vi "FTW-Logger-Construct.vi"(0 "Initialization Sequence":string, 5 "Logger Configuration":string, 11 "error in":errorcluster) -> (4 "FTW Logger":refnum<class "FTW-Logger-Core.lvclass">, 6 "Incoming Requests":refnum<event-registration>, 8 "Local Messages":refnum<event-registration>, 15 "error out":errorcluster)   [LabVIEW 2015, in "FTW-Logger-Core.lvclass"]
uses:
  FTW-Logger-Core.lvclass
  Message/Request/FTW-Message-IncomingRequest.lvclass
  Message/Base/FTW-Message.lvclass
  FTW-Logger-Core.lvclass/FTW-Logger-Core.ctl
  Error/FTW-ERR-NoErrorConstant.vi
  JSON/FTW-JSON-Core-LibraryFilepath.vi
  Error/FTW-ERR-ThrowError.vi
  JSON/core/FTW-JSON-Core-EncodingFlags.vi
  Reflection/FTW-Reflection-Type.vi
  CodeGen/JSON Deserialize/FTW-JSON-Core-GetFlattenedValue.vi
  CodeGen/JSON Deserialize/FTW-JSON-Deserialize.xnode
panel:
  # "Inputs"
  # "Outputs"
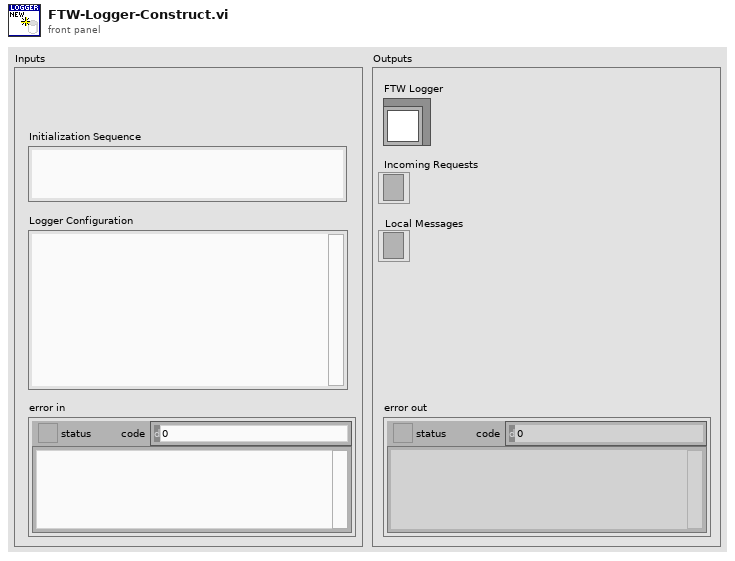
[diagram p1: front panel]
types:
  T1 = cluster{"ApplicationName":string, "LoggerName":string, "LoggerDirectory":path, "LoggerDiskThrashDelay":u32, "LoggerPublisher":string, "FilePeriod":string}
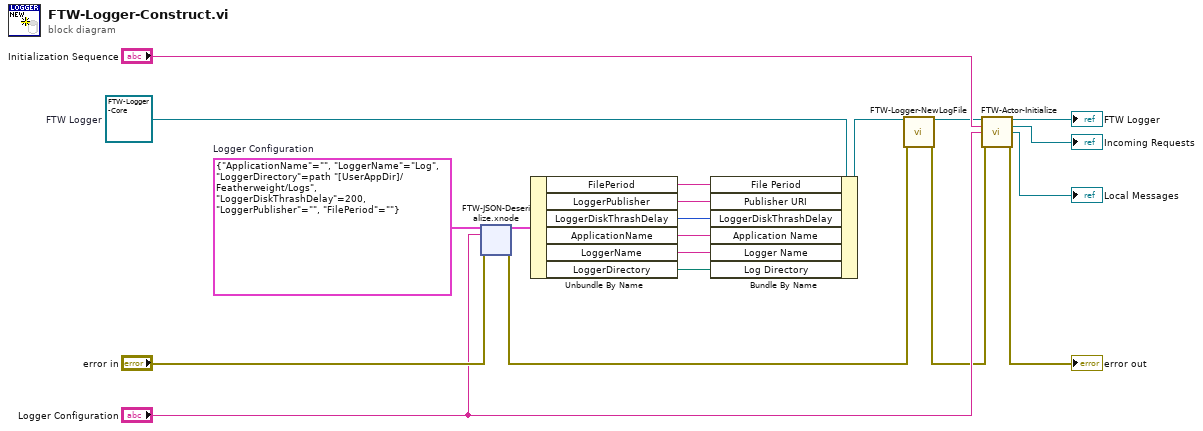
[diagram p0: block diagram]
diagram:
  w10 = T1 {"ApplicationName"="", "LoggerName"="Log", "LoggerDirectory"=path "[UserAppDir]/Featherweight/Logs", "LoggerDiskThrashDelay"=200, "LoggerPublisher"="", "FilePeriod"=""}  # Logger Configuration
  w20 = refnum<class "FTW-Logger-Core.lvclass"> refnum  # FTW Logger
  n1 = xnode "FTW-JSON-Deserialize.xnode"("Type and Defaults"=w10, "JSON String"="Logger Configuration", "error in"="error in") -> ("Values"=w11:T1, "error out"=w2:errorcluster)
  n2 = Unbundle By Name(w11) -> ("FilePeriod"=w5:string, "LoggerPublisher"=w9:string, "LoggerDiskThrashDelay"=w12:u32, "ApplicationName"=w7:string, "LoggerName"=w6:string, "LoggerDirectory"=w4:path)
  n3 = Bundle By Name(cluster=w20, "File Period"=w5, "Publisher URI"=w9, "LoggerDiskThrashDelay"=w12, "Application Name"=w7, "Logger Name"=w6, "Log Directory"=w4) -> (w13:refnum<class "FTW-Logger-Core.lvclass">)
  n4 = call "FTW-Logger-NewLogFile.vi"("FTW Logger"=w13, "error in"=w2) -> ("FTW Logger out"=w3:refnum<class "FTW-Logger-Core.lvclass">, "error out"=w1:errorcluster)  [unwired: 12 in]
  n5 = call-dynamic "FTW-Actor-Initialize.vi"("FTW Actor Instance Type"=w3, "Initialization Job Sequence"="Initialization Sequence", "Actor Instance Configuration"="Logger Configuration", "error in"=w1) -> ("FTW Actor Instance"=→"FTW Logger":refnum<class "FTW-Logger-Core.lvclass">, "Incoming Requests"=→"Incoming Requests":refnum<event-registration>, "Local Messages"=→"Local Messages":refnum<event-registration>, "error out"=→"error out":errorcluster)  [unwired: 8 in]
